vi "daqmx_trigger internally_test.impl.vi"(8 "error in":errorcluster) -> (0 "error out":errorcluster, 3 "task out":refnum<k21>)   [LabVIEW 2013]
uses:
  <vilib>/DAQmx/configure/trigger.llb/DAQmx Trigger.vi
  <vilib>/DAQmx/configure/trigger.llb/DAQmx Start Trigger (Digital Edge).vi
  <vilib>/DAQmx/configure/timing.llb/DAQmx Timing (Sample Clock).vi
  <vilib>/DAQmx/create/channels.llb/DAQmx Create Channel (AO-Voltage-Basic).vi
  <resource>/objmgr/daqmx.rc
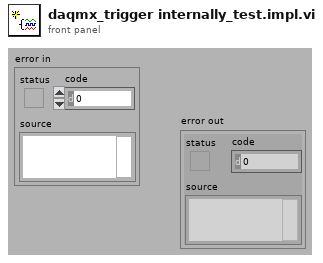
[diagram p1: front panel]
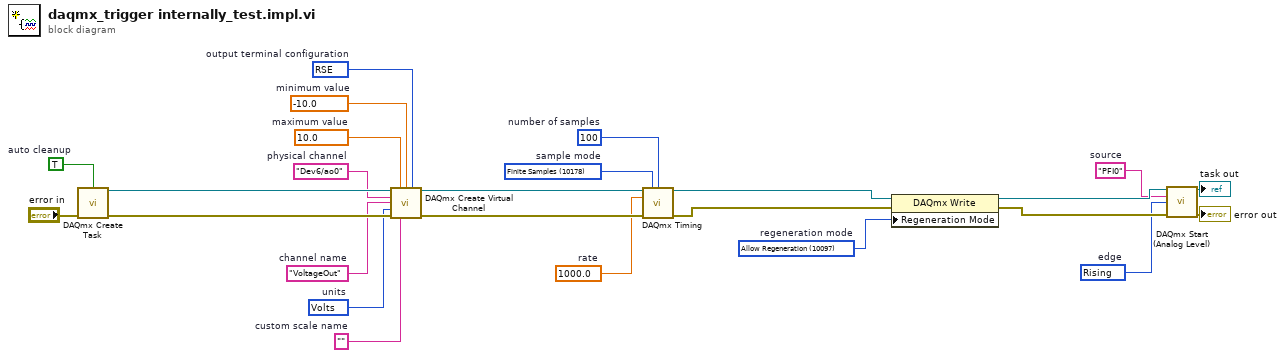
[diagram p0: block diagram]
diagram:
  w1 = 10280 items=["Rising"=10280, "Falling"=10171]  # edge
  w2 = "PFI0"  # source
  w6 = 10097 items=["Allow Regeneration"=10097, "Do Not Allow Regeneration"=10158]  # regeneration mode
  w9 = 10178 items=["Finite Samples"=10178, "Continuous Samples"=10123, "Hardware Timed Single Point"=12522]  # sample mode
  w10 = 100  # number of samples
  w11 = 1000.0  # rate
  w14 = 10083 items=["Default"=-1, "RSE"=10083, "Differential"=10106, "Pseudodifferential"=12529]  # output terminal configuration
  w15 = 10348 items=["Volts"=10348, "From Custom Scale"=10065]  # units
  w16 = "VoltageOut"  # channel name
  w18 = ""  # custom scale name
  w19 = -10.0  # minimum value
  w20 = 10.0  # maximum value
  w21 = "Dev6/ao0"  # physical channel
  w23 = TRUE  # auto cleanup
  n1 = call <vilib>:"DAQmx Create Task.vi"("auto cleanup"=w23, "error in"="error in") -> ("task out"=w22:refnum<k21>, "error out"=w24:errorcluster)  [unwired: 12 in]
  n2 = call-poly <vilib>:"DAQmx Create Virtual Channel.vi"("task in"=w22, "maximum value"=w20, "minimum value"=w19, "output terminal configuration"=w14, "physical channels"=w21, "name to assign"=w16, "units"=w15, "error in"=w24, "custom scale name"=w18) -> ("task out"=w12:refnum<k21>, "error out"=w17:errorcluster)  [unwired: 5 in]
  n3 = call-poly <vilib>:"DAQmx Timing.vi"("task/channels in"=w12, "sample mode"=w9, "samples per channel"=w10, "rate"=w11, "error in"=w17) -> ("task out"=w8:refnum<k21>, "error out"=w13:errorcluster)  [unwired: 9 in]
  n4 = property class="DAQmx Write"(reference=w8, error in=w13, "Regeneration Mode"=w6) -> (reference out=w3:refnum<k21>, error out=w7:errorcluster)
  n5 = call-poly "DAQmx Start (Analog Level).vi"("task/channels in"=w3, "source"=w2, "edge"=w1, "error in"=w7) -> ("task out"=→"task out":refnum<k21>, "error out"=→"error out":errorcluster)  [unwired: 10 in]
